vi "Initialise Sounds.vi"(8 "error in (no error)":errorcluster, 11 "Ship in":refnum<class "Ship.lvclass">) -> (0 "error out":errorcluster, 3 "Ship out":refnum<class "Ship.lvclass">)   [LabVIEW 2021, in "Ship.lvclass"]
uses:
  Ship.lvclass
  Ship.lvclass/Ship.ctl
  Resource Manager/Resource Manager.lvclass
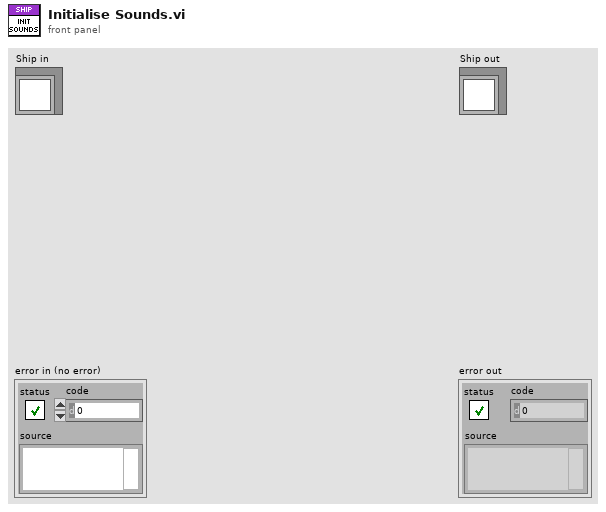
[diagram p1: front panel]
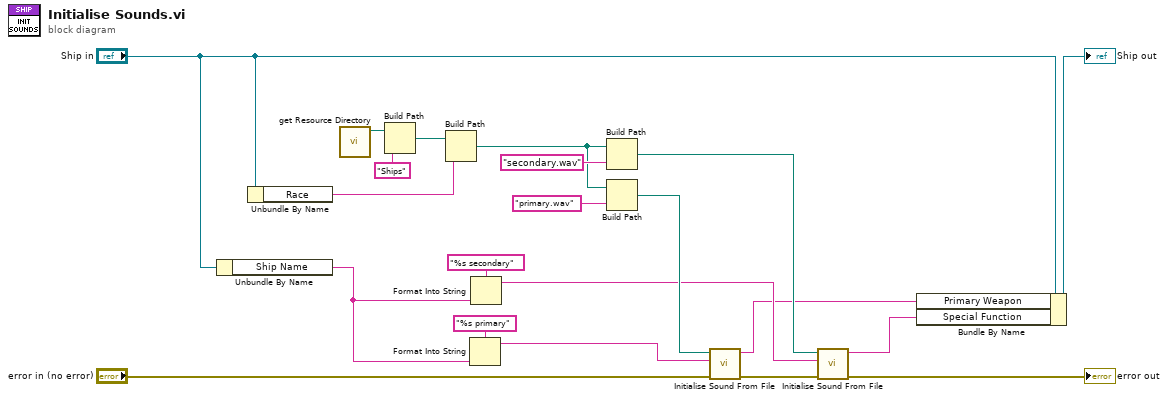
[diagram p0: block diagram]
diagram:
  n1 = Unbundle By Name("Ship in") -> ("Ship Name"=w1:string)
  n2 = Unbundle By Name("Ship in") -> ("Race"=w8:string)
  n3 = call "get Resource Directory.vi"() -> ("Resource Directory"=w19:path)  [unwired: 11 in]
  n4 = Build Path(base path=w19, name or relative path="Ships") -> (appended path=w21:path)
  n5 = Build Path(base path=w21, name or relative path=w8) -> (appended path=w3:path)
  n6 = Format Into String(format string="%s primary", w1) -> (resulting string=w6:string)  [unwired: 2 in, 1 out]
  n7 = Format Into String(format string="%s secondary", w1) -> (resulting string=w9:string)  [unwired: 2 in, 1 out]
  n8 = Build Path(base path=w3, name or relative path="secondary.wav" ("format string")) -> (appended path=w13:path)
  n9 = Build Path(base path=w3, name or relative path="primary.wav" ("format string")) -> (appended path=w14:path)
  n10 = call "Initialise Sound From File.vi"("error in (no error)"="error in (no error)", "Name"=w6, "File"=w14) -> ("error out"=w17:errorcluster, "Name In Cache"=w5:string)  [unwired: 7 in]
  n11 = call "Initialise Sound From File.vi"("error in (no error)"=w17, "Name"=w9, "File"=w13) -> ("error out"=→"error out":errorcluster, "Name In Cache"=w4:string)  [unwired: 7 in]
  n12 = Bundle By Name(cluster="Ship in", "Primary Weapon"=w5, "Special Function"=w4) -> (→"Ship out":refnum<class "Ship.lvclass">)
